vi "Start Client.vi"(8 "error in (no error)":errorcluster, 11 "LabVIEWHTTPClient_NET in":refnum<class "LabVIEWHTTPClient_NET.lvclass">) -> (0 "error out":errorcluster, 3 "LabVIEWHTTPClient_NET out":refnum<class "LabVIEWHTTPClient_NET.lvclass">)   [LabVIEW 2018, in "LabVIEWHTTPClient_NET.lvlib" / "LabVIEWHTTPClient_NET.lvclass"]
uses:
  LabVIEWHTTPClient_NET.lvclass
  LabVIEWHTTPClient_NET.lvclass/LabVIEWHTTPClient_NET.ctl
  System.Net.Http
  Accessors/Read NET_HttpClientHandler.vi
  Accessors/Write NET_HttpClient.vi
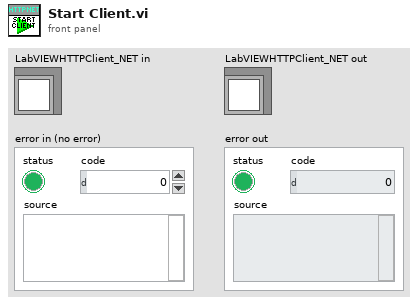
[diagram p1: front panel]
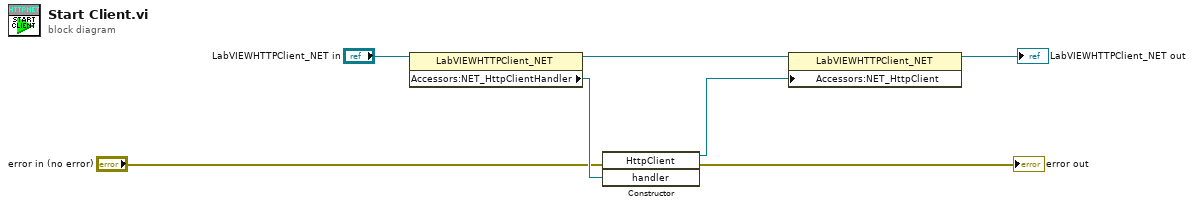
[diagram p0: block diagram]
diagram:
  n1 = property class="LabVIEWHTTPClient_NET"(reference="LabVIEWHTTPClient_NET in") -> (reference out=w5:refnum<class "LabVIEWHTTPClient_NET.lvclass">, "Accessors:NET_HttpClientHandler"=w4:refnum<k24>)  [unwired: 1 in, 1 out]
  n2 = constructor class="HttpClient"(error in="error in (no error)", "handler"=w4) -> (reference out=w7:refnum<k24>, error out=→"error out":errorcluster)  [unwired: 2 in, 2 out]
  n3 = property class="LabVIEWHTTPClient_NET"(reference=w5, "Accessors:NET_HttpClient"=w7) -> (reference out=→"LabVIEWHTTPClient_NET out":refnum<class "LabVIEWHTTPClient_NET.lvclass">)  [unwired: 1 in, 1 out]
